vi "Set Common Parameters.vi"(6 "fract diam":dbl=50.0 caption="FRACTURE DIAM (MM):", 7 "setpoint type":string, 8 "error in (no error)":errorcluster, 9 "test mech":enum32{"in vivo", "to fracture"}(radio), 10 "common test control":T1, 11 "IA Test Parameters in":refnum<class "IA Test Parameters.lvclass">) -> (0 "error out":errorcluster, 3 "IA Test Parameters out":refnum<class "IA Test Parameters.lvclass">)   [LabVIEW 2020]
uses:
  Controls/Common IA Test Control.ctl
  Parameter Class/IA Test Parameters.lvclass
  Parameter Class/IA Test Parameters.lvclass/IA Test Parameters.ctl
panel:
  # "TIME DELAY (SEC):"
  # "TEST TIME (SEC):"
  # "SAMPLING RATE (N/SEC):"
  # "DIAMETER ABORT (MM):"
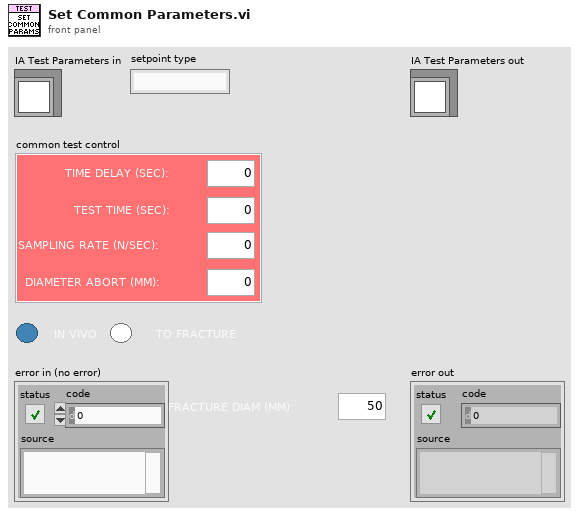
[diagram p1: front panel]
types:
  T1 = typedef "Common IA Test Control.ctl" = cluster{"time delay (sec)":dbl, "test time (sec)":dbl, "diameter abort (mm)":dbl, "sample rate (n/sec)":dbl}
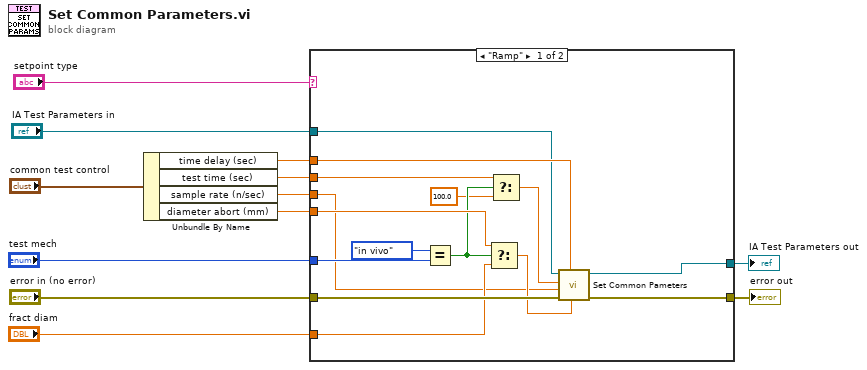
[diagram p0: block diagram]
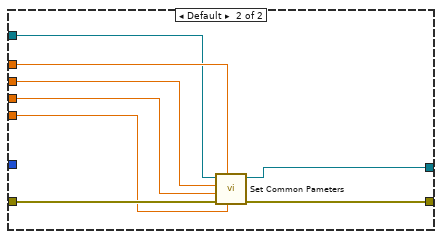
[diagram p2: hidden frame]
diagram:
  n1 = Unbundle By Name("common test control") -> ("time delay (sec)"=w12:dbl, "test time (sec)"=w7:dbl, "sample rate (n/sec)"=w6:dbl, "diameter abort (mm)"=w5:dbl)
  n2 = case shown="\"Ramp\"" "setpoint type" {
    tunnel: w12 -> [w15 w35]
    tunnel: [w13 w34] -> w10
    tunnel: [w26 w33] -> w9
    tunnel: "error in (no error)" -> [w27 w32]
    tunnel: w7 -> [w19 w31]
    tunnel: w6 -> [w16 w30]
    tunnel: w5 -> [w23 w29]
    tunnel: "IA Test Parameters in" -> [w14 w28]
    tunnel: "fract diam" -> [w22 _]
    tunnel: "test mech" -> [w25 _]
    frame "Ramp" {
      n3 = Equal?(x=enum32{"in vivo", "to fracture"}."in vivo", y=w25) -> (x = y?=w20:bool)
      n4 = Select(t=w23, s=w20, f=w22) -> (s? t:f=w21:dbl)
      n5 = Select(t=w19, s=w20, f=100.0) -> (s? t:f=w17:dbl)
      n6 = call "Set Common Pameters.vi"("diameter abort (mm)"=w21, "time delay (sec)"=w15, "error in (no error)"=w27, "sample rate (hz)"=w16, "test time (sec)"=w17, "IA Test Parameters in"=w14) -> ("error out"=w26:errorcluster, "IA Test Parameters out"=w13:refnum<class "IA Test Parameters.lvclass">)  [unwired: 4 in]
    }
    frame Default {
      n7 = call "Set Common Pameters.vi"("diameter abort (mm)"=w29, "time delay (sec)"=w35, "error in (no error)"=w32, "sample rate (hz)"=w30, "test time (sec)"=w31, "IA Test Parameters in"=w28) -> ("error out"=w33:errorcluster, "IA Test Parameters out"=w34:refnum<class "IA Test Parameters.lvclass">)  [unwired: 4 in]
    }
  }
  "IA Test Parameters out" <- w10
  "error out" <- w9
